vi "Append Last Packet.vi"(4 "Movement Correction":bool, 6 "Repeat Scan":i32, 7 "MAC Address":string, 10 "Packets":string[](array[string]), 11 "AOL_Globals":T1={"Imaging Protocol"=enum."AOL Z-Stack", "Number of POI"=0, "Number of Miniscans"=0, "Number of Trials"=0, "Number of Cycles "=0, "# Averaged Frames"=0, "Laser power (%)"=0, "Pockels (V)"=0.0, "Acquisition Length (sec)"=0.0, "Fill time (us)"=0.0, "POI Dwell time (us)"=0.0, "Miniscan Dwell time per pixel (us)"=0.0, "PMT 1"=0.0, "PMT 2"=0.0, "Back Apperture (mA)"=0.0, "Frame Size"=0, "Center Frequency"=0.0, "Field of View (norm)"=0.0, "DwellTime (us)"=0.0, "Wavelength (nm)"=0.0, "Zoom"=0.0, "AOL Z"=0.0, "AOL Mode"=enum."Raster", "GridXY"=0.0, "GridZ"=0.0, "TriggerPeriod (sec)"=0.0, "Number of Pixels in Miniscan"=0, "Experiment folder path"=path "", "X centre"=0.0, "Y centre"=0.0, "Angle (degrees)"=0.0, "Plane Mode"=0, "Threshold"=[], "Regenerate Chirps"=FALSE, "Rectangle ROI length (pixels)"=0, "Rectangle ROI height (pixels)"=0, "AOD fill"=4900, "StartupDelay"=0, "Samples Wait after Trigger"=5080, "Slip Cycle"=600000, "Add Cycle"=TRUE, "Functional Mode"=enum."Point", "Z Start"=0.0, "Z Stop"=0.0, "# Planes"=0, "Total Pixels"=0, "Variable Miniscan Pixels"=[], "Use Variable Length"=FALSE, "Use Variable Resolution"=FALSE, "Laser power (%) at Z Start"=0, "Laser power (%) at Z Stop"=0, "Ref Z Step"=0, "Ref Dwell Time (us)"=0.0, "Field of View (um)"=175.0} {"Plane Mode" items=["XY Plane", "XZ Plane", "YZ Plane", "arbitraryplane"]; "Frame Size" items=["100X100"=100, "128X128"=128, "200X200"=200, "256X256"=256, "512X512"=512, "1024x1024"=1024, "2048x2048"=2048]; "Back Apperture (mA)" format="%#.6g"; "Pockels (V)" format="%#.6g"; "PMT 2" format="%#.6g"; "PMT 1" format="%#.6g"; "Angle (degrees)" format="%#.6g"; "POI Dwell time (us)" format="%#.6g"}) -> (0 "Repeat":i32, 2 "HexPackets":string[](array[string]), 3 "Total Packets":i32)   [LabVIEW 2020]
uses:
  Typedefs/Controls/AOL_Globals.ctl
  Typedefs/Imaging Protocols enum.ctl
  Typedefs/Frame Size.ctl
  Typedefs/AOL modes.ctl
  Typedefs/Plane Mode.ctl
  Typedefs/Functional Mode.ctl
panel:
  out "String":string
  out "*(type *) &x":string
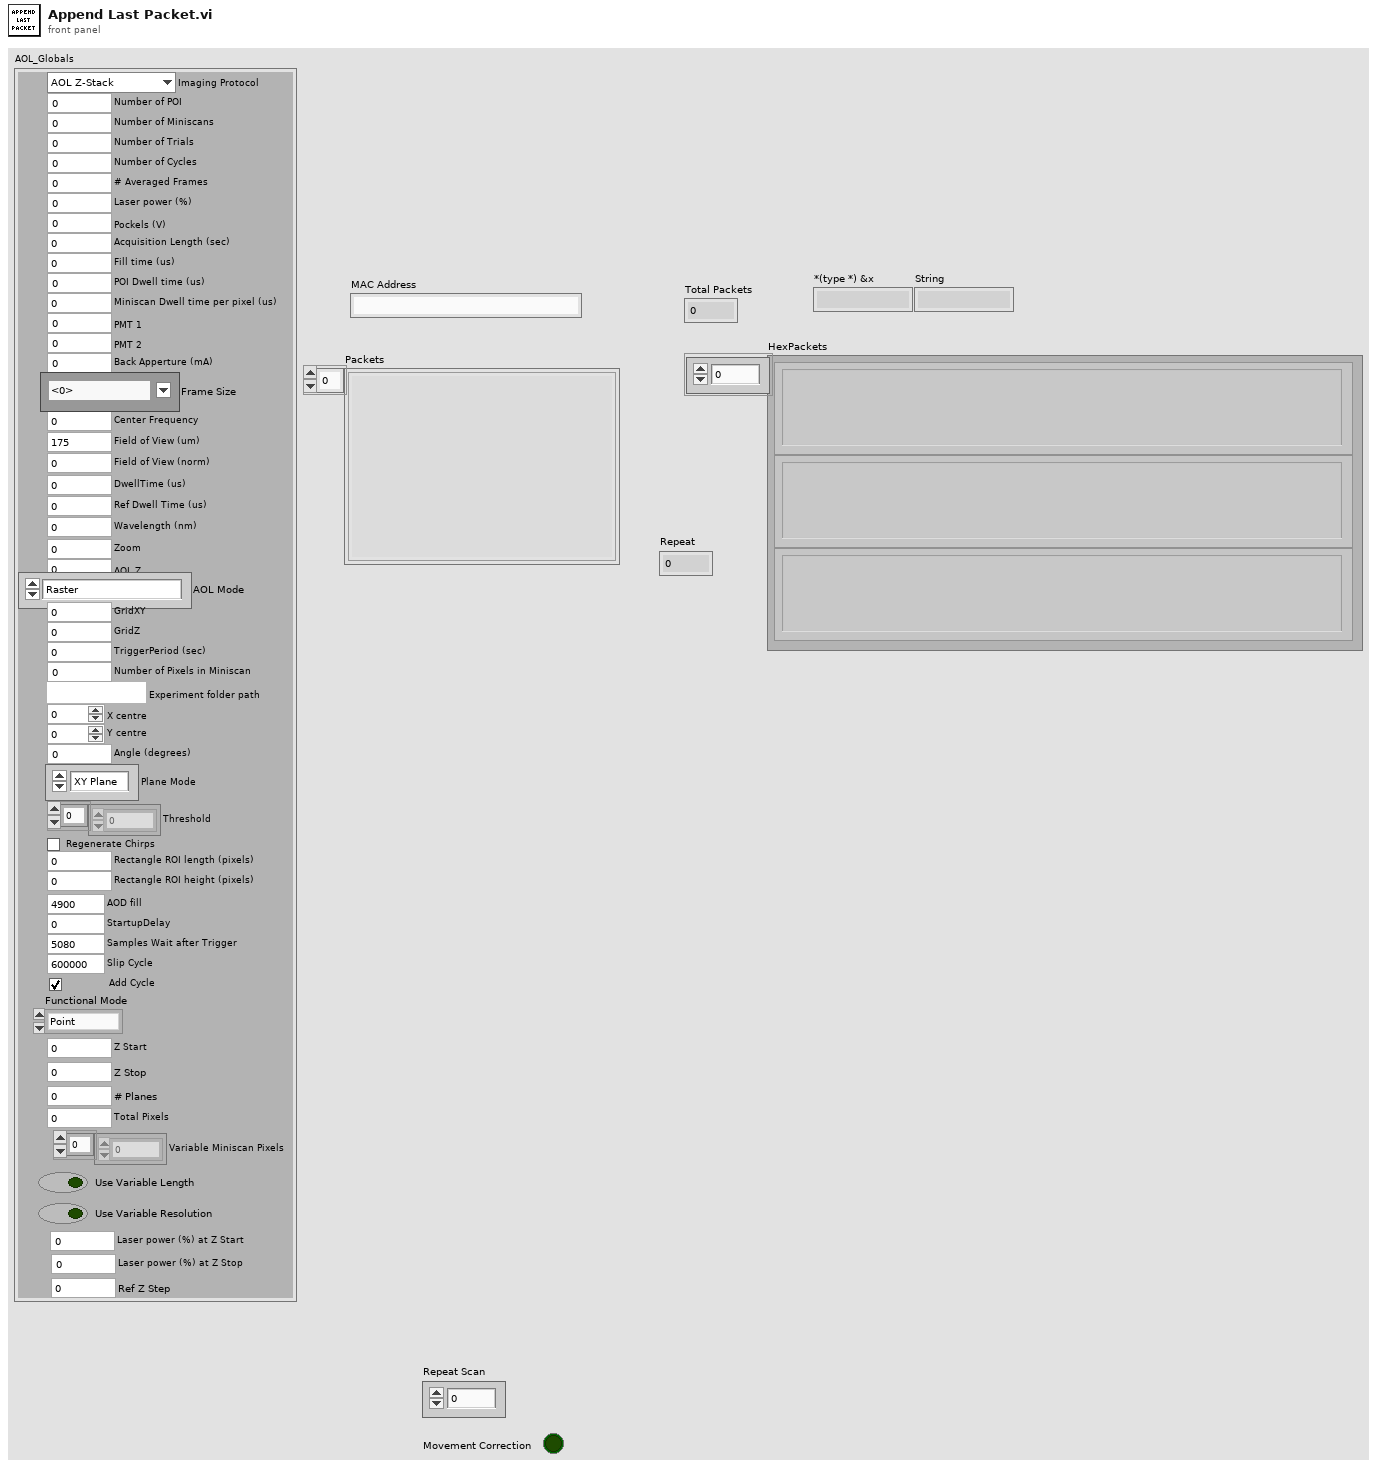
[diagram p1: front panel]
types:
  T1 = typedef "AOL_Globals.ctl" = cluster{"Imaging Protocol":T2, "Number of POI":u16, "Number of Miniscans":u16, "Number of Trials":u16, "Number of Cycles ":u64, "# Averaged Frames":u16, "Laser power (%)":u8, "Pockels (V)":dbl, "Acquisition Length (sec)":dbl, "Fill time (us)":dbl, "POI Dwell time (us)":dbl, "Miniscan Dwell time per pixel (us)":dbl, "PMT 1":dbl, "PMT 2":dbl, "Back Apperture (mA)":dbl, "Frame Size":T3, "Center Frequency":dbl, "Field of View (norm)":dbl, "DwellTime (us)":dbl, "Wavelength (nm)":dbl, "Zoom":dbl, "AOL Z":dbl, "AOL Mode":T4, "GridXY":dbl, "GridZ":dbl, "TriggerPeriod (sec)":dbl, "Number of Pixels in Miniscan":u16, "Experiment folder path":path, "X centre":dbl, "Y centre":dbl, "Angle (degrees)":dbl, "Plane Mode":T5, "Threshold":u16[], "Regenerate Chirps":bool, "Rectangle ROI length (pixels)":u16, "Rectangle ROI height (pixels)":u16, "AOD fill":u16, "StartupDelay":i32, "Samples Wait after Trigger":u16, "Slip Cycle":u32, "Add Cycle":bool, "Functional Mode":T6, "Z Start":dbl, "Z Stop":dbl, "# Planes":i32, "Total Pixels":i32, "Variable Miniscan Pixels":u16[], "Use Variable Length":bool, "Use Variable Resolution":bool, "Laser power (%) at Z Start":u8, "Laser power (%) at Z Stop":u8, "Ref Z Step":i8, "Ref Dwell Time (us)":dbl, "Field of View (um)":dbl}
  T2 = typedef "Imaging Protocols enum.ctl" = enum16{"AOL Z-Stack", "Motor Z Stack", "Functional Acquisition", "Single Plane Acquisition", "Volume Acquisition", "Live Imaging", "Live Plane Imaging", "Live Volume Imaging"}
  T3 = typedef "Frame Size.ctl" = u16
  T4 = typedef "AOL modes.ctl" = enum16{"Raster", "Structural", "Pointing", "Mini Scan", "Alignment"}
  T5 = typedef "Plane Mode.ctl" = u16
  T6 = typedef "Functional Mode.ctl" = enum16{"Point", "Line", "Patch", "Plane", "Volume"}
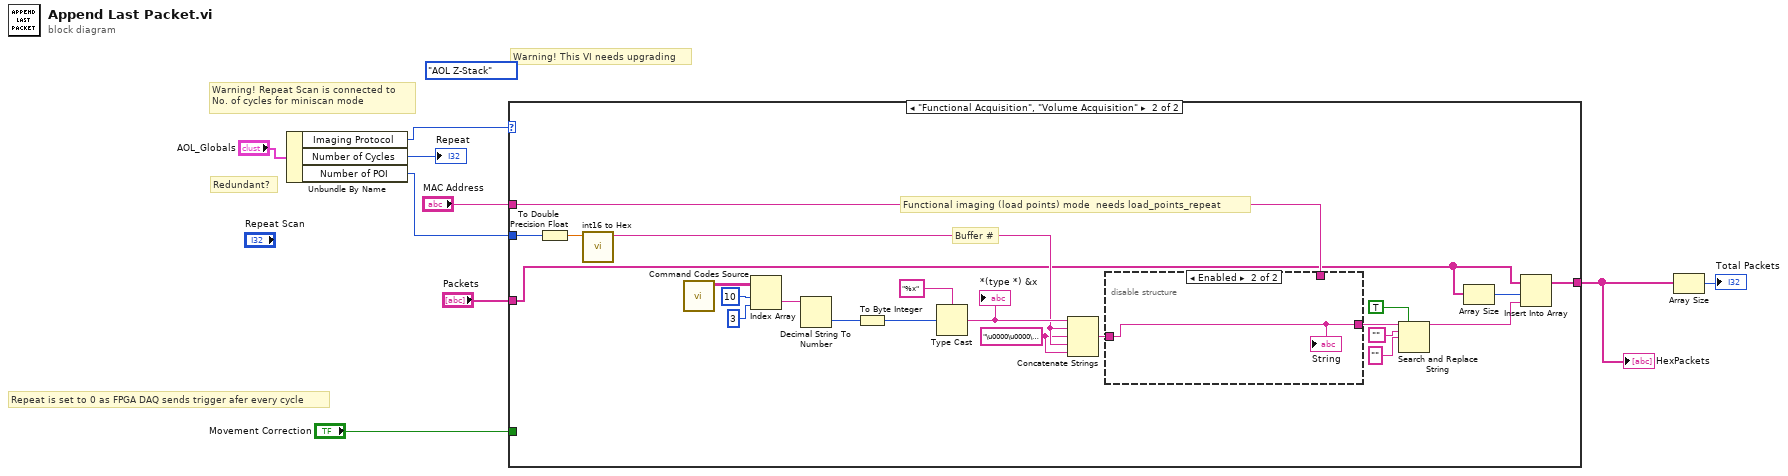
[diagram p0: block diagram]
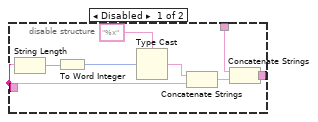
[diagram p3: hidden frame]
diagram:
  (unwired) Imaging_Protocols_enum."AOL Z-Stack" ("Imaging Protocol")
  # "Repeat is set to 0 as FPGA DAQ sends trigger afer every cycle"
  # "Warning! This VI needs upgrading"
  # "Redundant?"
  # "Warning! Repeat Scan is connected to \nNo. of cycles for miniscan mode"
  n1 = Unbundle By Name("AOL_Globals") -> ("Imaging Protocol"=w5:T2, "Number of Cycles"=→"Repeat":u64, "Number of POI"=w1:u16)
  n2 = case shown="\"Functional Acquisition\", \"Volume Acquisition\"" w5 {
    tunnel: [w10 w18] -> w6
    tunnel: "Packets" -> [w10 w12]
    tunnel: "MAC Address" -> [_ w17]
    tunnel: "Movement Correction" -> [_ _]
    tunnel: w1 -> [_ w15]
    frame "Live Imaging", Default {
    }
    frame "Functional Acquisition", "Volume Acquisition" {
      w13 = "\u0000\u0000\u0000\u0000" ("string")
      # "Buffer #"
      # "Functional imaging (load points) mode  needs load_points_repeat"
      n3 = To Double Precision Float(number=w15) -> (double precision float=w16:dbl)
      n4 = call "int16 to Hex.vi"("number"=w16) -> ("Hex string"=w14:string)  [unwired: 10 in]
      n5 = call "Command Codes Source.vi"() -> ("Commands for FPGA"=w28:string[][])  [unwired: 11 in]
      n6 = Index Array(array=w28, index (row)=10 ("disabled index (row)"), index (col)=3 ("disabled index (col)")) -> (element=w22:string)
      n7 = Decimal String To Number(string=w22) -> (number=w24:i32)  [unwired: 2 in, 1 out]
      n8 = To Byte Integer(number=w24) -> (8bit integer=w23:i8)
      n9 = Type Cast(type="%x", x=w23) -> (*(type *) &x=w21:string)
      "*(type *) &x" <- w21
      n10 = Concatenate Strings(w21, w14, w13, w14, w13) -> (w20:string)
      n11 = disable-structure shown="Enabled" {
        disable-tunnel: [w36 w41] -> w32
        disable-tunnel: w20 -> [w34 w41]
        disable-tunnel: w17 -> [w33 _]
        frame Disabled {
          n12 = String Length(string=w34) -> (length=w37:i32)
          n13 = To Word Integer(number=w37) -> (16bit integer=w35:i16)
          n14 = Type Cast(type="%x", x=w35) -> (*(type *) &x=w39:string)
          n15 = Concatenate Strings(w39, w34) -> (w40:string)
          n16 = Concatenate Strings(w33, w40) -> (w36:string)
        }
        frame Enabled {
          "String" <- w41
        }
      }
      n17 = Search and Replace String(replace all?=TRUE ("replace all? (F)"), input string=w32, search string="", replace string="" ("replace string (\"\")")) -> (result string=w19:string)  [unwired: 4 in, 3 out]
      n18 = Array Size(array=w12) -> (size(s)=w11:i32)
      n19 = Insert Into Array(array=w12, index=w11, new element=w19) -> (w18:string[])
    }
  }
  "HexPackets" <- w6
  n20 = Array Size(array=w6) -> (size(s)=→"Total Packets":i32)
